vi "RTS Build Default Headers.vi"(8 "Error In":errorcluster, 11 "Chamber Data in":string[][](array[string])) -> (0 "Error Out":errorcluster, 3 "New Header Save Array":T1[](array[typedef]))   [LabVIEW 2018]
uses:
  Washer DOE/Type Definitions/DOE Data Save Modifier.ctl
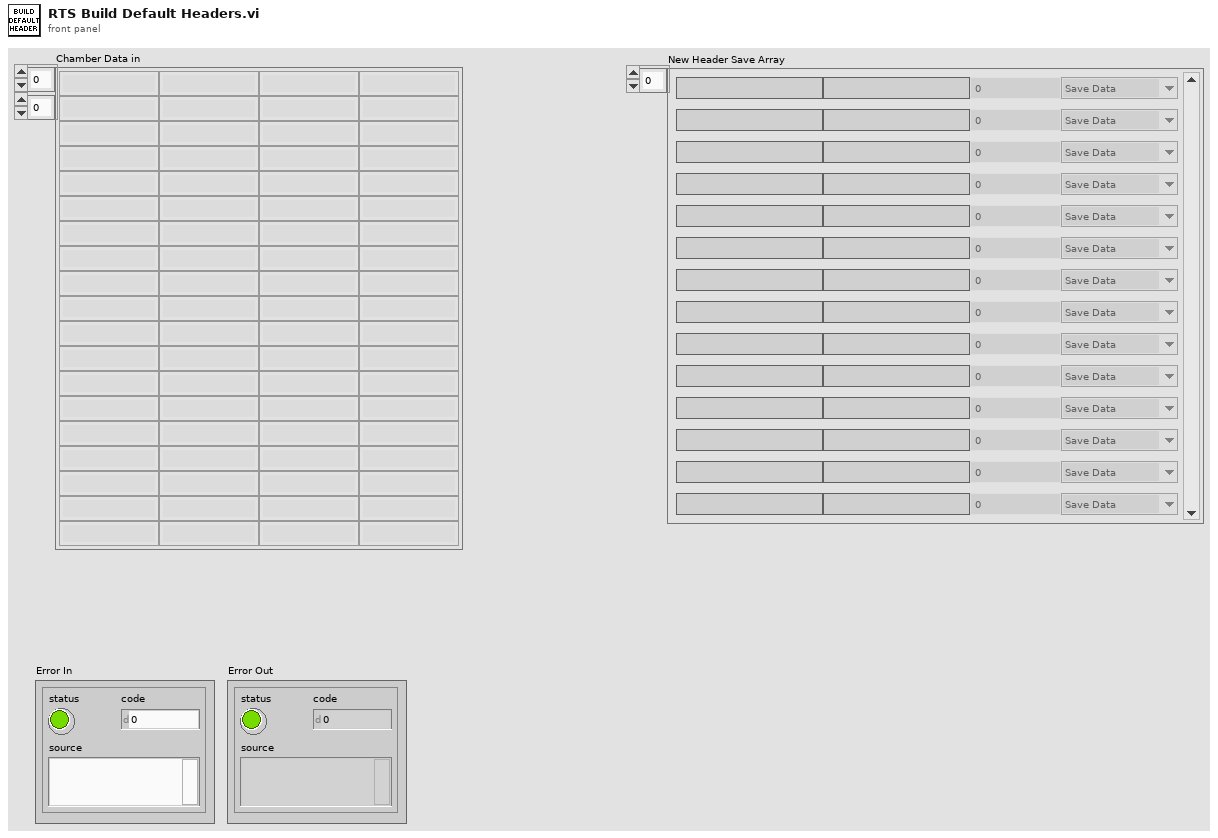
[diagram p1: front panel]
types:
  T1 = typedef "DOE Data Save Modifier.ctl" = cluster{"Name":string, "Title":string, "Save Status":enum16{"Save Data", "Don't Save Data"}, "Group":u8, "Field":u8}
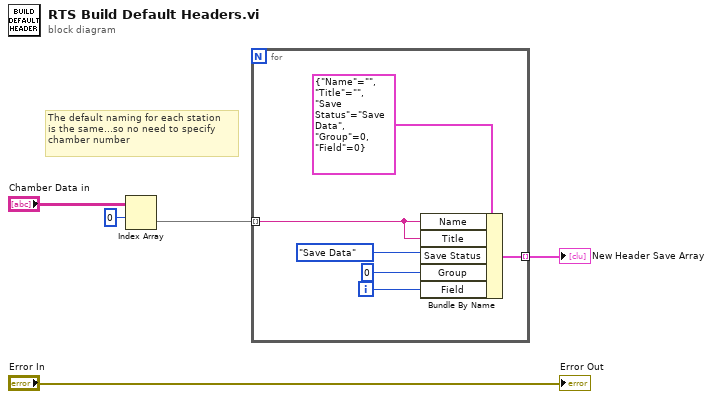
[diagram p0: block diagram]
diagram:
  # "The default naming for each station\nis the same...so no need to specify\nchamber number"
  n1 = Index Array(array="Chamber Data in", index (row)=0) -> (element=w2:string[])  [unwired: 1 in]
  n2 = for {
    tunnel: w2 -> [w6] mode=indexing
    tunnel: [w7] -> w1 mode=indexing
    i -> [w10]
    n3 = Bundle By Name(cluster=T1 {"Name"="", "Title"="", "Save Status"=enum."Save Data", "Group"=0, "Field"=0} ("Cluster"), "Name"=w6, "Title"=w6, "Save Status"=enum16{"Save Data", "Don't Save Data"}."Save Data", "Group"=u8 0, "Field"=w10) -> (w7:T1)
  }
  "New Header Save Array" <- w1
  "Error Out" <- "Error In"
